vi "OP500ZP_ADJ.vi"(8 "errin":errorcluster caption="entrée d'erreur (pas d'erreur)", 10 "BT3562A":string(combo) caption="Nom de ressource VISA") -> (0 "errout":errorcluster caption="sortie d'erreur", 2 "ADJ?":bool)   [LabVIEW 2020]
uses:
  <vilib>/Instr/_visa.llb/VISA Configure Serial Port (Instr).vi
  <instrlib>/HIOKI BT356X Series/HIOKI BT356X Series.lvlib
panel:
  out "POSTadj":string
  out "PRETadj":string
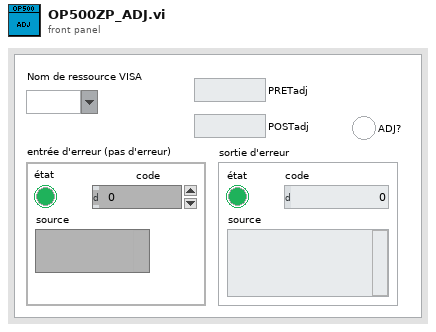
[diagram p1: front panel]
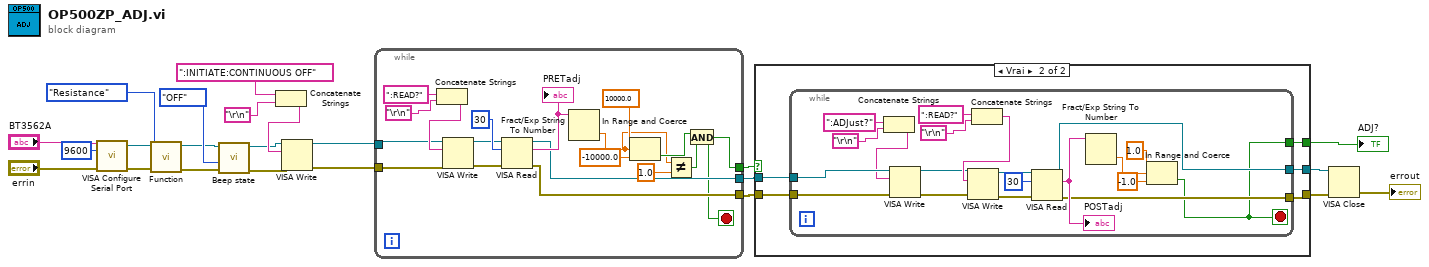
[diagram p0: block diagram]
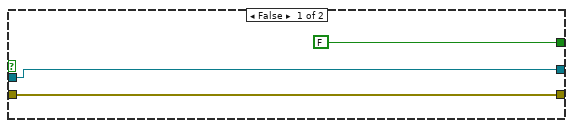
[diagram p2: hidden frame]
diagram:
  n1 = call-poly "VISA Configure Serial Port"("VISA resource name"="BT3562A", "baud rate (9600)"=u32 9600, "error in (no error)"="errin") -> ("VISA resource name out"=w7:refnum<visa-resource-name>, "error out"=w8:errorcluster)  [unwired: 11 in]
  n2 = call <instrlib>:"Function.vi"("error in (no error)"=w8, "Function set"=enum16{"RV", "Resistance", "Voltage"}."Resistance", "VISA session"=w7) -> ("error out"=w2:errorcluster, "dup VISA session"=w4:refnum<visa-resource-name>)  [unwired: 6 in, 1 out]
  n3 = call <instrlib>:"Beep state.vi"("error in (no error)"=w2, "Beep set"=enum16{"ON", "OFF"}."OFF", "VISA session"=w4) -> ("error out"=w1:errorcluster, "dup VISA session"=w3:refnum<visa-resource-name>)  [unwired: 6 in, 1 out]
  n4 = Concatenate Strings(":INITIATE:CONTINUOUS OFF" ("buffer d'écriture"), "\r\n") -> (w13:string)
  n5 = VISA Write(VISA resource name=w3, write buffer=w13, error in (no error)=w1) -> (VISA resource name out=w9:refnum<visa-resource-name>, error out=w10:errorcluster)  [unwired: 1 out]
  n6 = while {
    tunnel: [w26] -> w16
    tunnel: [w34] -> w15
    tunnel: [w33] -> w14
    tunnel: w10 -> [w25]
    tunnel: w9 -> [w24]
    stop <- w26 stop-if-true
    n7 = Concatenate Strings(":READ?" ("buffer d'écriture"), "\r\n") -> (w37:string)
    n8 = VISA Write(VISA resource name=w24, write buffer=w37, error in (no error)=w25) -> (VISA resource name out=w40:refnum<visa-resource-name>, error out=w36:errorcluster)  [unwired: 1 out]
    n9 = VISA Read(VISA resource name=w40, byte count=u32 30 ("nombre d'octets"), error in (no error)=w36) -> (VISA resource name out=w33:refnum<visa-resource-name>, read buffer=w35:string, error out=w34:errorcluster)  [unwired: 1 out]
    "PRETadj" <- w35
    n10 = Fract/Exp String To Number(string=w35) -> (number=w28:dbl)  [unwired: 3 in, 1 out]
    n11 = In Range and Coerce(upper limit=10000.0 ("limite supérieure"), x=w28, lower limit=-10000.0 ("limite inférieure")) -> (In Range?=w30:bool)  [unwired: 1 out]
    n12 = Not Equal?(x=w28, y=1.0) -> (x != y?=w27:bool)
    n13 = And(x=w30, y=w27) -> (x .and. y?=w26:bool)
  }
  n14 = case shown="Vrai" w16 {
    tunnel: [FALSE w45] -> w23
    tunnel: [w43 w46] -> w22
    tunnel: [w44 w47] -> w21
    tunnel: w15 -> [w44 w49]
    tunnel: w14 -> [w43 w48]
    frame False {
    }
    frame True {
      n15 = while {
        tunnel: w49 -> [w69]
        tunnel: w48 -> [w68]
        tunnel: [w52] -> w47
        tunnel: [w51] -> w46
        tunnel: [w50] -> w45
        stop <- w50 stop-if-true
        n16 = Concatenate Strings(":ADJust?" ("buffer d'écriture"), "\r\n") -> (w65:string)
        n17 = VISA Write(VISA resource name=w68, write buffer=w65, error in (no error)=w69) -> (VISA resource name out=w61:refnum<visa-resource-name>, error out=w60:errorcluster)  [unwired: 1 out]
        n18 = Concatenate Strings(":READ?" ("buffer d'écriture"), "\r\n") -> (w62:string)
        n19 = VISA Write(VISA resource name=w61, write buffer=w62, error in (no error)=w60) -> (VISA resource name out=w59:refnum<visa-resource-name>, error out=w58:errorcluster)  [unwired: 1 out]
        n20 = VISA Read(VISA resource name=w59, byte count=u32 30 ("nombre d'octets"), error in (no error)=w58) -> (VISA resource name out=w51:refnum<visa-resource-name>, read buffer=w53:string, error out=w52:errorcluster)  [unwired: 1 out]
        "POSTadj" <- w53
        n21 = Fract/Exp String To Number(string=w53) -> (number=w54:dbl)  [unwired: 3 in, 1 out]
        n22 = In Range and Coerce(upper limit=1.0 ("limite supérieure"), x=w54, lower limit=-1.0 ("limite inférieure")) -> (In Range?=w50:bool)  [unwired: 1 out]
      }
    }
  }
  "ADJ?" <- w23
  n23 = VISA Close(VISA resource name=w22, error in (no error)=w21) -> (error out=→"errout":errorcluster)
